vi "Vision Research Phantom Series PhFile PhReadCineImage.vi"(1 "CH in":u32, 2 "BITMAPINFOHEADER":T1, 3 "ImageNumber":i32, 4 "Options(0)":u32, 5 "Error In (no error)":errorcluster, 8 "Simulate? (False)":bool) -> (15 "CH out":u32, 16 "pPixel16":u16[](array[numeric]), 17 "pPixel8":u8[](array[numeric]), 19 "Error Out":errorcluster)   [LabVIEW 2013, in "VRI.lvlib"]
doc: "PhReadCineImage\nCH(in) Handle of the file cine.\nImageNumber(in) The number of the cine image that is to be read.\nOptions(in) -Reading options. Used now for multi-head camera cines to identify the head number.\n Possible values:\n \" 0 to 3 - get cine image from head 0..3\n \" -1 - get cine image from all heads\n Options parameter is ignored for single head camera cines.\n\npPixel(out) Image pixels.\n\nReturn ERR_Ok - The operation has succeeded. \n\nComments:\nThis function returns the image pixels for the specified image of the cine. \nYou can get the BITMAPINFOHEADER structure using PhGetCineBMIH. \n\nWritten by:\nBLOOMY CONTROLS, INC\nWINDSOR, CT 06095, USA\n860-298-9925\nwww.bloomy.com\nV1.0.0\nMay, 2004"
uses:
  VRI.lvlib
  Projects/SDK/32-bit/Vision Research Phantom Series Labview Driver/Phantom DLLs/PhFile.dll
  _Type Defs/PhFile InfName.ctl
  _Type Defs/BITMAPINFOHEADER.ctl
panel:
  # "For instructions on the use of this VI, press Ctrl+H to display the help window and move the mouse over the icon, controls, and indicators"
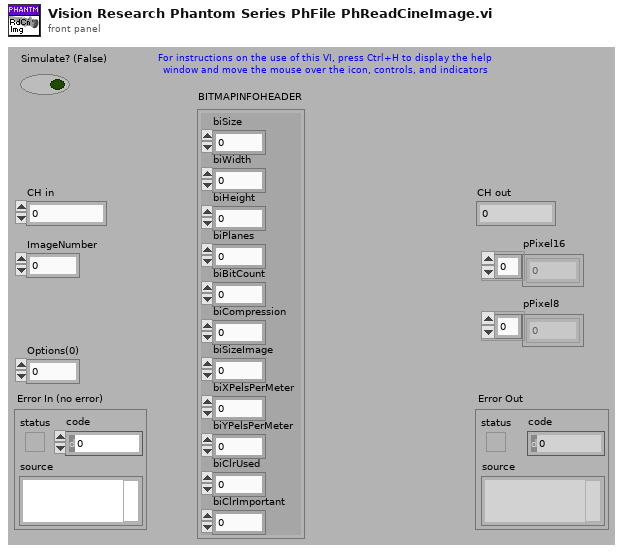
[diagram p1: front panel]
types:
  T1 = typedef "VRI.lvlib/BITMAPINFOHEADER.ctl" = cluster{"biSize":u32, "biWidth":i32, "biHeight":i32, "biPlanes":u16, "biBitCount":u16, "biCompression":u32, "biSizeImage":u32, "biXPelsPerMeter":i32, "biYPelsPerMeter":i32, "biClrUsed":u32, "biClrImportant":u32}
  T2 = typedef "VRI.lvlib/PhFile InfName.ctl" = u32
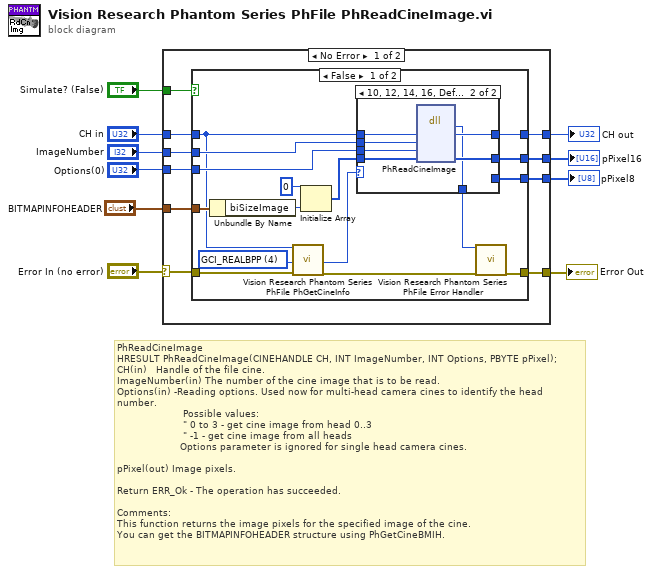
[diagram p0: block diagram]
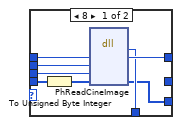
[diagram p2: hidden frame]
diagram:
  # "PhReadCineImage\nHRESULT PhReadCineImage(CINEHANDLE CH, INT ImageNumber, INT Options, PBYTE pPixel);\nCH(in)  \tHandle of the file cine.\nImageNumber(in) The number of the cine image that is to be read.\nOptions(in) -Reading options. Used now for multi-head camera cines to identify the head number.\n                      Possible values:\n                      \"\t0 to 3 - get cine image from head 0..3\n                      \"\t-1 - get cine image from all heads\n                     Options parameter is ignored for single head camera cines.\n\npPixel(out) Image pixels.\n\nReturn\tERR_Ok - The operation has succeeded. \n\nComments:\nThis function returns the image pixels for the specified image of the cine. \nYou can get the BITMAPINFOHEADER structure using PhGetCineBMIH."
  n1 = case shown="No Error" "Error In (no error)" {
    selector: "Error In (no error)" -> [w20 w55]
    tunnel: [w19 w55] -> w9
    tunnel: "Simulate? (False)" -> [w18 _]
    tunnel: "ImageNumber" -> [w17 _]
    tunnel: "CH in" -> [w16 w54]
    tunnel: [w15 w54] -> w5
    tunnel: [w14 _] -> w4
    tunnel: "Options(0)" -> [w13 _]
    tunnel: "BITMAPINFOHEADER" -> [w12 _]
    tunnel: [w11 _] -> w1
    frame No Error {
      n2 = case shown="False" w18 {
        tunnel: w20 -> [w27 w53]
        tunnel: [w28 w53] -> w19
        tunnel: w17 -> [w35 _]
        tunnel: w16 -> [w23 w52]
        tunnel: [w34 w52] -> w15
        tunnel: [w31 _] -> w14
        tunnel: w13 -> [w32 _]
        tunnel: w12 -> [w30 _]
        tunnel: [w21 _] -> w11
        frame False {
          w24 = T2 4 items=["GCI_CFA"=0, "GCI_FRAMERATE"=1, "GCI_EXPOSURE"=2, "GCI_AUTOEXPOSURE"=3, "GCI_REALBPP"=4, "GCI_CAMERASERIAL"=5, "GCI_HEADSERIAL0"=6, "GCI_HEADSERIAL1"=7, "GCI_HEADSERIAL2"=8, "GCI_HEADSERIAL3"=9, "GCI_TRIGTIMESEC"=10, "GCI_TRIGTIMEFR"=11, "GCI_ISFILECINE"=12, "GCI_IS16BPPCINE"=13, "GCI_ISCOLORCINE"=14, "GCI_ISMULTIHEADCINE"=15, "GCI_EXPOSURENS"=16, "GCI_EDREXPOSURENS"=17, "GCI_FRAMEDELAYNS"=19, "GCI_FROMFILETYPE"=20, "GCI_COMPRESSION"=21, "GCI_CAMERAVERSION"=22, "GCI_ROTATE"=23, "GCI_IMWIDTH"=24, "GCI_IMHEIGHT"=25, "GCI_IMWIDTHACQ"=26, "GCI_IMHEIGHTACQ"=27, "GCI_POSTTRIGGER"=28, "GCI_IMAGECOUNT"=29, "GCI_TOTALIMAGECOUNT"=30, "GCI_TRIGFRAME"=31, "GCI_AUTOEXPLEVEL"=32, "GCI_AUTOEXPTOP"=33, "GCI_AUTOEXPLEFT"=34, "GCI_AUTOEXPBOTTOM"=35, "GCI_AUTOEXPRIGHT"=36, "GCI_RECORDINGTIMEZONE"=37, "GCI_FRPSTEPS"=100, "GCI_FRP1X"=101, "GCI_FRP1Y"=102, "GCI_FRP2X"=103, "GCI_FRP2Y"=104, "GCI_FRP3X"=105, "GCI_FRP3Y"=106, "GCI_FRP4X"=107, "GCI_FRP4Y"=108] ("InfName")
          n3 = Unbundle By Name(w30) -> ("biSizeImage"=w29:u32)
          n4 = call "Vision Research Phantom Series PhFile PhGetCineInfo.vi"("CH in"=w23, "InfName"=w24, "Error In (no error)"=w27) -> ("pInfVal out"=w22:i32, "Error Out"=w26:errorcluster)  [unwired: 15 out]
          n5 = Initialize Array(u16 0, w29) -> (w33:u16[])
          n6 = case shown="10, 12, 14, 16, Default" w22 {
            tunnel: w35 -> [w43 w51]
            tunnel: w23 -> [w44 w50]
            tunnel: [w42 w49] -> w34
            tunnel: w33 -> [w39 w48]
            tunnel: w32 -> [w41 w47]
            tunnel: [_ w46] -> w31
            tunnel: [w38 w45] -> w25
            tunnel: [w37 _] -> w21
            frame 8 {
              n7 = To Unsigned Byte Integer(number=w39) -> (unsigned 8bit integer=w40:u8[])
              n8 = dll-call lib="C:/Projects/SDK/32-bit/Vision Research Phantom Series Labview Driver/Phantom DLLs/PhFile.dll" fn="PhReadCineImage"("CH"=w44, "ImageNumber"=w43, "Options"=w41, "pPixel"=w40) -> ("HRESULT"=w38:i32, "CH"=w42:u32, "pPixel"=w37:u8[])  [unwired: 5 in, 2 out]
            }
            frame 10, 12, 14, 16, Default {
              n9 = dll-call lib="C:/Projects/SDK/32-bit/Vision Research Phantom Series Labview Driver/Phantom DLLs/PhFile.dll" fn="PhReadCineImage"("CH"=w50, "ImageNumber"=w51, "Options"=w47, "pPixel"=w48) -> ("HRESULT"=w45:i32, "CH"=w49:u32, "pPixel"=w46:u16[])  [unwired: 5 in, 2 out]
            }
          }
          n10 = call "Vision Research Phantom Series PhFile Error Handler.vi"("Error Code (0)"=w25, "Error In (no error)"=w26) -> ("Error Out"=w28:errorcluster)  [unwired: 17 out]
        }
        frame True {
          # "It looks as though the dlls can provide simulated data so this case may not have to be used"
        }
      }
    }
    frame Error {
    }
  }
  "Error Out" <- w9
  "pPixel16" <- w4
  "CH out" <- w5
  "pPixel8" <- w1
